vi "Agilent DCPower and Keithley Scope.vi"() -> ()   [LabVIEW 2021]
doc: "Configures the power supply's output range on a channel, configures the DC voltage level, channel appears at the output connector and takes a measurement on the output signal and returns the measured value."
uses:
  <instrlib>/Agilent N6700 Series/Agilent N6700 Series.lvlib
  <instrlib>/Tektronix MSO5X Series/Tektronix MSO5X Series.lvlib
panel:
  in  "Tettronix Scope":refnum<visa-resource-name>
  out "Interpolation Ratio":dbl
  out "Timebase Duration (s)":dbl
  out "Division Number":i32
  in  "Control Type":i32(ring) items=["Horizontal Scale", "Record Length"]
  in  "Sample Rate":dbl=3125000000.0
  in  "Maximum Record Length":dbl=250000000.0 format="%#_6e"
  in  "error in":errorcluster {"code" format="%.0x"}
  out "error out":errorcluster {"code" format="%.0x"}
  in  "Current Limit":dbl=1.0 format="%^.3e"
  in  "Behavior":i32(ring) items=["Regulatory Limit", "Trip Limit"]
  out "Voltage Measurement":dbl format="%^.3e"
  in  "Voltage Level":dbl=5.0 format="%^.3e"
  in  "Voltage Range":dbl=10.0 format="%^.3e"
  in  "Agilent SMUChannel":string="1"
  in  "Agilent SMU":refnum<visa-resource-name>
  # "Agilent N6700 DC Power Supply"
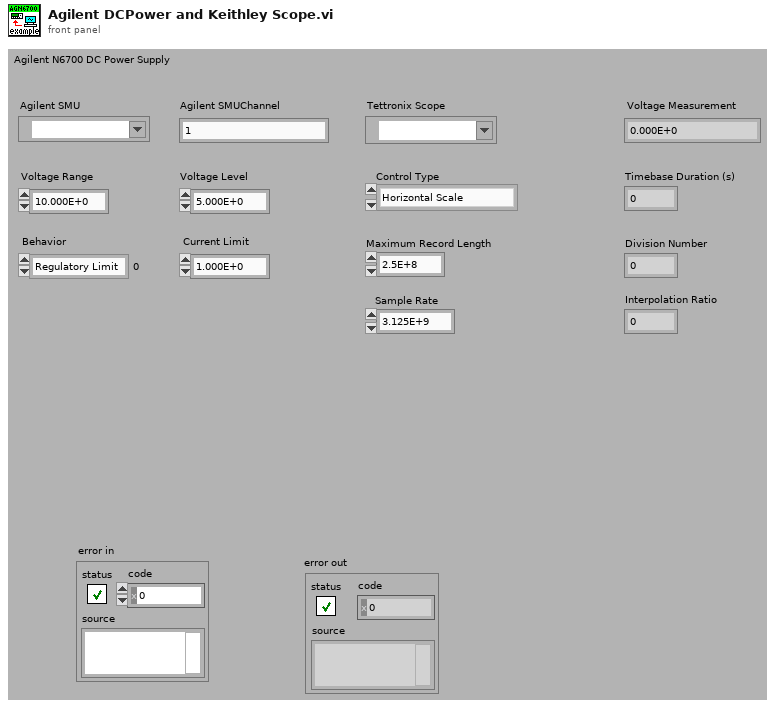
[diagram p1: front panel]
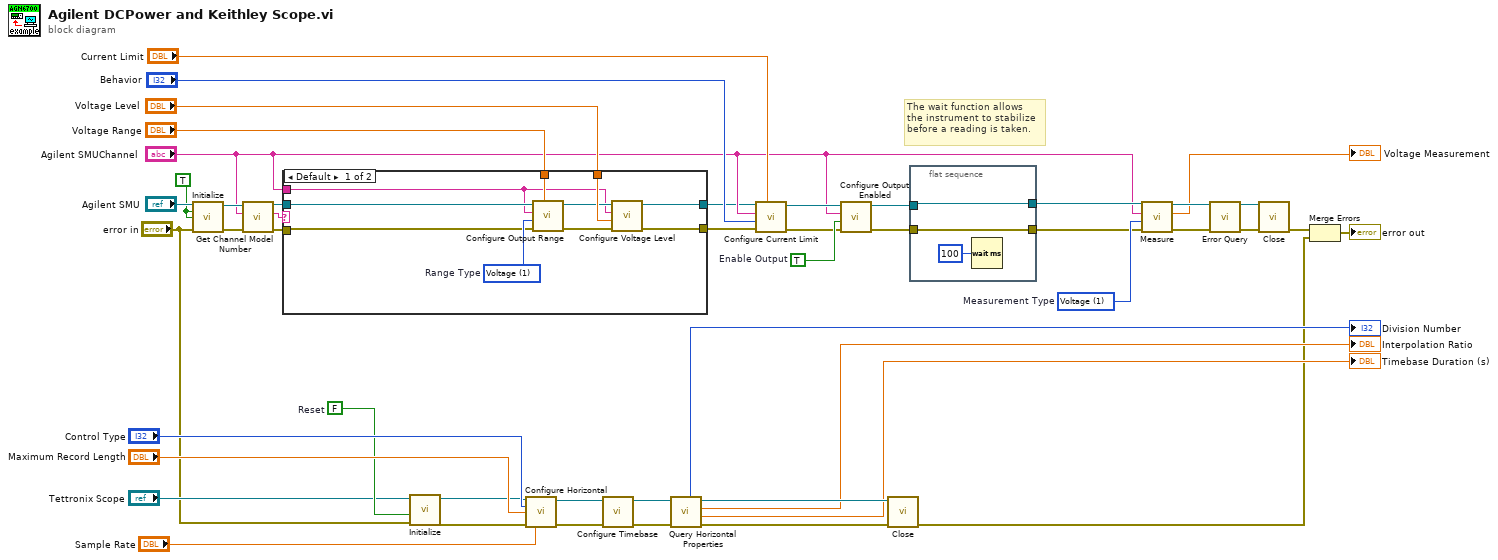
[diagram p0: block diagram]
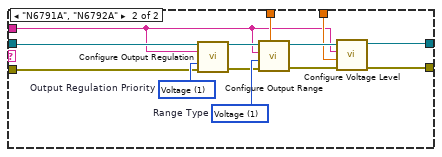
[diagram p2: hidden frame]
diagram:
  w5 = FALSE  # Reset
  w38 = TRUE ("Reset? (T: Yes)")
  w39 = 1 items=["Voltage"=1, "Current"=0]  # Measurement Type
  w40 = TRUE  # Enable Output
  # "The wait function allows \nthe instrument to stabilize\nbefore a reading is taken."
  n1 = call <instrlib>:"Initialize.vi"("VISA resource name"="Agilent SMU", "ID Query? (T: Yes)"=w38, "Reset? (T: Yes)"=w38, "error in (no error)"="error in") -> ("VISA resource name out"=w29:refnum<visa-resource-name>, "error out"=w28:errorcluster)  [unwired: 10 in]
  n2 = call <instrlib>:"Get Channel Model Number.vi"("error in (no error)"=w28, "Channel Name (1)"="Agilent SMUChannel", "VISA resource name"=w29) -> ("error out"=w26:errorcluster, "Model Number"=w25:string, "VISA resource name out"=w27:refnum<visa-resource-name>)  [unwired: 6 in]
  n3 = case shown="Default" w25 {
    tunnel: "Voltage Range" -> [w54 w70]
    tunnel: "Agilent SMUChannel" -> [w48 w60]
    tunnel: w27 -> [w56 w65]
    tunnel: w26 -> [w55 w64]
    tunnel: "Voltage Level" -> [w52 w61]
    tunnel: [w50 w58] -> w22
    tunnel: [w49 w59] -> w21
    frame Default {
      w57 = 1 items=["Voltage"=1, "Current"=0]  # Range Type
      n4 = call <instrlib>:"Configure Output Range.vi"("Range (0.0)"=w54, "error in (no error)"=w55, "Range Type (1: Voltage)"=w57, "Channel Name (1)"=w48, "VISA resource name"=w56) -> ("error out"=w53:errorcluster, "VISA resource name out"=w51:refnum<visa-resource-name>)  [unwired: 5 in]
      n5 = call <instrlib>:"Configure Voltage Level.vi"("error in (no error)"=w53, "Level  (0.0 volts)"=w52, "Channel Name (1)"=w48, "VISA resource name"=w51) -> ("error out"=w50:errorcluster, "VISA resource name out"=w49:refnum<visa-resource-name>)  [unwired: 6 in]
    }
    frame "N6791A", "N6792A" {
      w66 = 1 items=["Voltage"=1, "Current"=0]  # Output Regulation Priority
      w69 = 1 items=["Voltage"=1, "Current"=0]  # Range Type
      n6 = call <instrlib>:"Configure Output Regulation.vi"("VISA resource name"=w65, "Channel Name (1)"=w60, "Output Regulation Priority (1: Voltage)"=w66, "error in (no error)"=w64) -> ("VISA resource name out"=w68:refnum<visa-resource-name>, "error out"=w67:errorcluster)  [unwired: 10 in]
      n7 = call <instrlib>:"Configure Output Range.vi"("Range (0.0)"=w70, "error in (no error)"=w67, "Range Type (1: Voltage)"=w69, "Channel Name (1)"=w60, "VISA resource name"=w68) -> ("error out"=w62:errorcluster, "VISA resource name out"=w63:refnum<visa-resource-name>)  [unwired: 5 in]
      n8 = call <instrlib>:"Configure Voltage Level.vi"("error in (no error)"=w62, "Level  (0.0 volts)"=w61, "Channel Name (1)"=w60, "VISA resource name"=w63) -> ("error out"=w58:errorcluster, "VISA resource name out"=w59:refnum<visa-resource-name>)  [unwired: 6 in]
    }
  }
  n9 = call <instrlib>:"Initialize.vi"("error in (no error)"="error in", "Reset (True)"=w5, "VISA resource name"="Tettronix Scope") -> ("error out"=w7:errorcluster, "VISA resource name out"=w6:refnum<visa-resource-name>)  [unwired: 7 in]
  n10 = call <instrlib>:"Configure Horizontal.vi"("VISA resource name"=w6, "Control Type (0: Horizontal Scale)"="Control Type", "Maximum Record Length (2.5E+8)"="Maximum Record Length", "error in (no error)"=w7, "Sample Rate (3.125E+9)"="Sample Rate") -> ("VISA resource name out"=w16:refnum<visa-resource-name>, "error out"=w17:errorcluster)  [unwired: 9 in]
  n11 = call <instrlib>:"Configure Timebase.vi"("error in (no error)"=w17, "VISA resource name"=w16) -> ("error out"=w18:errorcluster, "VISA resource name out"=w19:refnum<visa-resource-name>)  [unwired: 8 in]
  n12 = call <instrlib>:"Query Horizontal Properties.vi"("error in (no error)"=w18, "VISA resource name"=w19) -> ("error out"=w15:errorcluster, "Timebase Duration (s)"=→"Timebase Duration (s)":dbl, "Interpolation Ratio"=→"Interpolation Ratio":dbl, "VISA resource name out"=w14:refnum<visa-resource-name>, "Division Number"=→"Division Number":i32)  [unwired: 5 in]
  n13 = call <instrlib>:"Configure Current Limit.vi"("Limit (0.0 amps)"="Current Limit", "error in (no error)"=w22, "Behavior (0: Regulatory Limit)"="Behavior", "Channel Name (1)"="Agilent SMUChannel", "VISA resource name"=w21) -> ("error out"=w37:errorcluster, "VISA resource name out"=w36:refnum<visa-resource-name>)  [unwired: 5 in]
  n14 = call <instrlib>:"Configure Output Enabled.vi"("error in (no error)"=w37, "Enable Output (False)"=w40, "Channel Name (1)"="Agilent SMUChannel", "VISA resource name"=w36) -> ("error out"=w30:errorcluster, "VISA resource name out"=w33:refnum<visa-resource-name>)  [unwired: 6 in]
  n15 = call <instrlib>:"Close.vi"("error in (no error)"=w15, "VISA resource name"=w14) -> ("error out"=w2:errorcluster)  [unwired: 9 in]
  n16 = flat-sequence {
    tunnel: w33 -> [w73]
    tunnel: [w73] -> w32
    tunnel: [w71] -> w31
    tunnel: w30 -> [w71]
    frame #0 {
      n17 = Wait (ms)(milliseconds to wait=u32 100) -> ()  [unwired: 1 out]
    }
  }
  n18 = call <instrlib>:"Measure.vi"("error in (no error)"=w31, "Measurement Type (1: Voltage)"=w39, "Channel Name (1)"="Agilent SMUChannel", "VISA resource name"=w32) -> ("error out"=w47:errorcluster, "Measurement"=→"Voltage Measurement":dbl, "VISA resource name out"=w44:refnum<visa-resource-name>)  [unwired: 5 in]
  n19 = call <instrlib>:"Error Query.vi"("VISA resource name"=w44, "error in (no error)"=w47) -> ("VISA resource name out"=w45:refnum<visa-resource-name>, "error out"=w46:errorcluster)  [unwired: 10 in, 2 out]
  n20 = call <instrlib>:"Close.vi"("VISA resource name"=w45, "error in (no error)"=w46) -> ("error out"=w20:errorcluster)  [unwired: 13 in]
  n21 = Merge Errors(w20, w2) -> (→"error out":errorcluster)
